vi "wind turbine speed measurement.vi"() -> ()   [LabVIEW 2018]
doc: "I. Description:\nThis example demonstrates how to count digital events on a Counter Input Channel. The Initial Count, Count Direction, and Edge are all configurable. \n\nEdges are counted on the counter's default input terminal (see I/O Connections for more information), but could easily be modified to count edges on a PFI or RTSI line.\n\nII. Instructions for Running:\n1. Select the Physical Channel which corresponds to the counter you want to count edges on the DAQ device.\n2. Enter the Initial Count, Count Direction, and measurement Edge to specify how you want the counter to count. Additionally, you can change the input terminal where events are counted using the channel property node.\nNote: Use the Gen Dig Pulse Train-Continuous example to verify that you are counting correctly on the DAQ device.\n\nIII. Block Diagram Steps:\n1. Create a Counter Input channel to Count Events. The Edge parameter is used to determine if the counter will increment on rising or falling edges.\n2. Call the Start VI to arm the counter and begin counting. The counter will be preloaded with the Initial Count.\n3. The counter will be continually polled until the Stop button is pressed on the front panel.\n4. Call the Clear Task VI to clear the Task.\n5. Use the popup dialog box to display an error if any.\n\nIV. I/O Connections Overview:\nThe counter will count edges on the input terminal of the counter specified in the Physical Channel I/O control.\n\nIn this example the counter will count edges on the default input terminal on ctr0.\n\nFor more information on the default counter input and output terminals for your device, open the NI-DAQmx Help, and refer to Counter Signal Connections found under the Device Considerations book in the table of contents."
uses:
  <vilib>/Utility/error.llb/DialogType.ctl
  <vilib>/DAQmx/read.llb/DAQmx Read (Counter U32 1Chan 1Samp).vi
  <vilib>/DAQmx/create/channels.llb/DAQmx Create Channel (CI-Count Edges).vi
  <vilib>/DAQmx/miscellaneous.llb/DAQmx Fill In Error Info.vi
panel:
  in  "calibration factor":dbl=1.0
  out "Waveform Chart":dbl(graph)=866.6145905006338
  out "period":dbl=0.00033283233642578125
  out "revs per min":dbl=704.5645589565383
  out "revs per sec":dbl=11.736389684813753
  out "counts per sec":dbl=3004.515759312321
  in  "counter":tag="Dev2/ctr0"
  in  "stop":bool
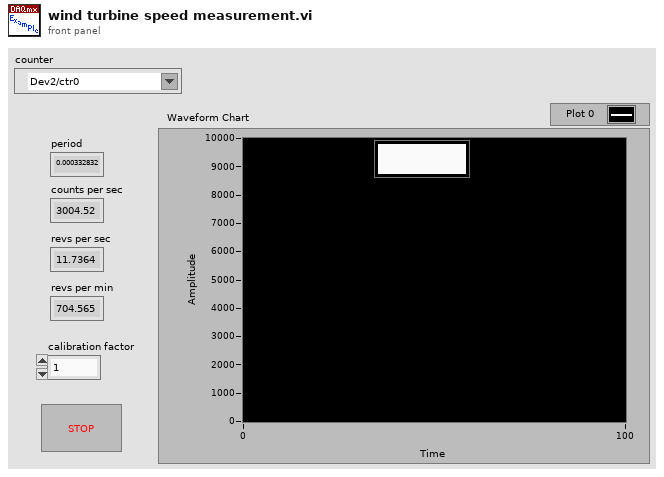
[diagram p1: front panel]
types:
  T1 = typedef "DialogType.ctl" = u16
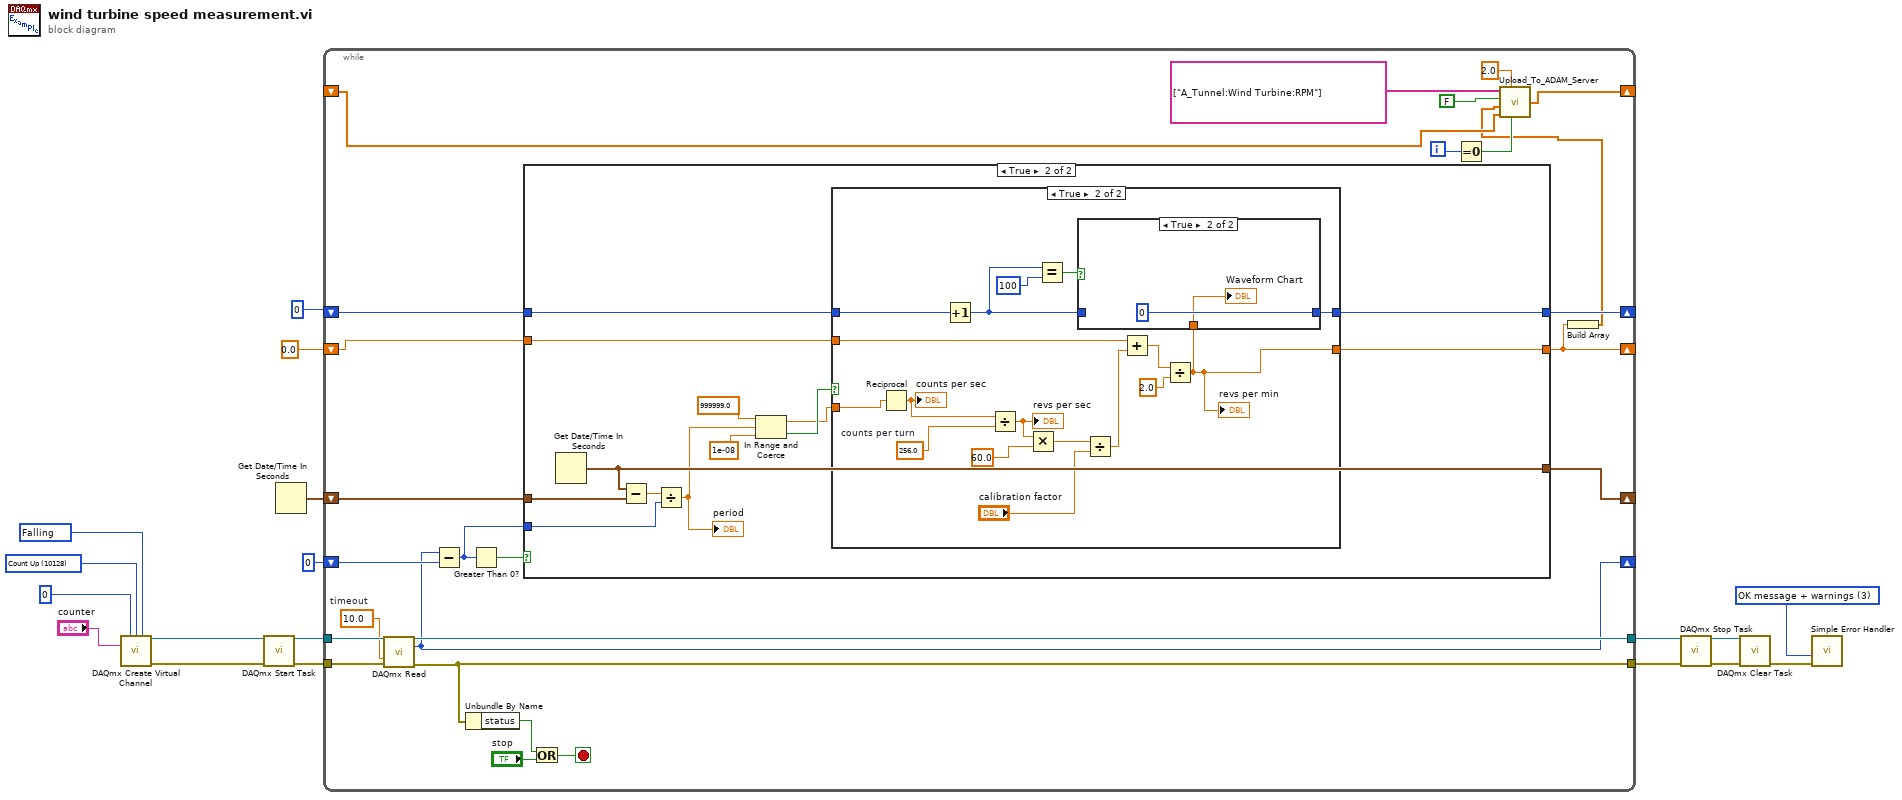
[diagram p0: block diagram]
diagram:
  w15 = 10171 items=["Rising"=10280, "Falling"=10171] ("Edge")
  w13 = 10128 items=["Count Up"=10128, "Count Down"=10124, "Externally Controlled"=10326] ("Count Direction")
  w9 = T1 3 items=["no dialog", "OK message", "continue or stop message", "OK message + warnings", "continue/stop + warnings"] ("type of dialog (OK msg:1)")
  n1 = call-poly <vilib>:"DAQmx Create Virtual Channel.vi"("initial count"=u32 0 ("Initial Count"), "count direction"=w13, "edge"=w15, "counter"="counter") -> ("task out"=w17:refnum<k21>, "error out"=w18:errorcluster)  [unwired: 10 in]
  n2 = call <vilib>:"DAQmx Start Task.vi"("task/channels in"=w17, "error in"=w18) -> ("task out"=w10:refnum<k21>, "error out"=w12:errorcluster)  [unwired: 12 in]
  n3 = Get Date/Time In Seconds() -> (seconds since 1Jan1904=w4:timestamp)
  n4 = while {
    tunnel: w12 -> [w44]
    tunnel: [w40] -> w7
    tunnel: w10 -> [w39]
    tunnel: [w38] -> w8
    shift-right: [w33] -> _
    shift-left: u32 0 ("data") -> [w34]
    shift-right: [w36] -> _
    shift-left: w4 -> [w35]
    shift-right: [w20] -> _
    shift-left: 0.0 ("lower limit") -> [w30]
    shift-right: [w28] -> _
    shift-left: 0 ("lower limit") -> [w29]
    shift-right: [w24] -> _
    shift-left: _ -> [w21]
    i -> [w23]
    stop <- w43 stop-if-true
    w37 = 10.0  # timeout
    n5 = call-poly <vilib>:"DAQmx Read.vi"("task/channels in"=w39, "timeout"=w37, "error in"=w44) -> ("task out"=w38:refnum<k21>, "data"=w33:u32, "error out"=w40:errorcluster)  [unwired: 10 in]
    n6 = Subtract(x=w33, y=w34) -> (x-y=w31:u32)
    n7 = Unbundle By Name(w40) -> ("status"=w41:bool)
    n8 = Greater Than 0?(x=w31) -> (x > 0?=w32:bool)
    n9 = case shown="True" w32 {
      tunnel: [w47 w60] -> w36
      tunnel: w35 -> [w47 w59]
      tunnel: w31 -> [_ w57]
      tunnel: [w46 w51] -> w20
      tunnel: w30 -> [w46 w50]
      tunnel: w29 -> [w45 w49]
      tunnel: [w45 w48] -> w28
      frame False {
      }
      frame True {
        n10 = Get Date/Time In Seconds() -> (seconds since 1Jan1904=w60:timestamp)
        n11 = Subtract(x=w60, y=w59) -> (x-y=w58:dbl)
        n12 = Divide(x=w58, y=w57) -> (x/y=w52:dbl)
        "period" <- w52
        n13 = In Range and Coerce(upper limit=999999.0, x=w52, lower limit=1e-08) -> (coerced(x)=w53:dbl, In Range?=w54:bool)
        n14 = case shown="True" w54 {
          tunnel: w53 -> [_ w79]
          tunnel: [w62 w63] -> w51
          tunnel: w50 -> [w62 w71]
          tunnel: w49 -> [w61 w68]
          tunnel: [w61 w64] -> w48
          frame False {
          }
          frame True {
            w77 = 256.0  # counts per turn
            n15 = Reciprocal(x=w79) -> (1/x=w78:dbl)
            "counts per sec" <- w78
            n16 = Increment(x=w68) -> (x+1=w65:i32)
            n17 = Divide(x=w78, y=w77) -> (x/y=w76:dbl)
            "revs per sec" <- w76
            n18 = Multiply(x=w76, y=60.0 ("counts per turn")) -> (x*y=w74:dbl)
            n19 = Equal?(x=w65, y=100 ("lower limit")) -> (x = y?=w67:bool)
            n20 = Divide(x=w74, y="calibration factor") -> (x/y=w72:dbl)
            n21 = Add(x=w71, y=w72) -> (x+y=w70:dbl)
            n22 = Divide(x=w70, y=2.0 ("counts per turn")) -> (x/y=w63:dbl)
            "revs per min" <- w63
            n23 = case shown="True" w67 {
              tunnel: w65 -> [w80 _]
              tunnel: [w80 0 ("lower limit")] -> w64
              tunnel: w63 -> [_ w81]
              frame False {
              }
              frame True {
                "Waveform Chart" <- w81
              }
            }
          }
        }
      }
    }
    n24 = Or(x=w41, y="stop") -> (x .or. y?=w43:bool)
    n25 = Equal To 0?(x=w23) -> (x = 0?=w22:bool)
    n26 = Build Array(w20) -> (w19:dbl[])
    n27 = call "Upload_To_ADAM_Server.vi"("First Loop"=w22, "Averaging Period (s)"=2.0, "Shift In"=w21, "Channel Values"=w19, "Give Variance"=FALSE, "Channel Names"=string[] ["A_Tunnel:Wind Turbine:RPM"]) -> ("Shift Out"=w24:dbl[])
  }
  n28 = call <vilib>:"DAQmx Stop Task.vi"("task/channels in"=w8, "error in"=w7) -> ("task out"=w5:refnum<k21>, "error out"=w6:errorcluster)  [unwired: 12 in]
  n29 = call <vilib>:"DAQmx Clear Task.vi"("task in"=w5, "error in"=w6) -> ("error out"=w11:errorcluster)  [unwired: 13 in]
  n30 = call <vilib>:"Simple Error Handler.vi"("type of dialog (OK msg:1)"=w9, "error in (no error)"=w11) -> ()  [unwired: 3 in, 5 out]
